vi "GPIOs.vi"(8 "error in (no error)":errorcluster, 11 "I2C in":refnum<class "I2C.lvclass">) -> (0 "error out":errorcluster, 1 "SDA GPIO":T1, 2 "SCL GPIO":T1, 3 "I2C out":refnum<class "I2C.lvclass">)   [LabVIEW 2020, in "CTI.lvlib" / "I2C.lvclass"]
uses:
  I2C.lvclass
  GPIO Number.ctl
  I2C.lvclass/I2C.ctl
  GPIO/GPIO.lvclass/GPIO.ctl
  GPIO/GPIO.lvclass
  CTI.lvlib
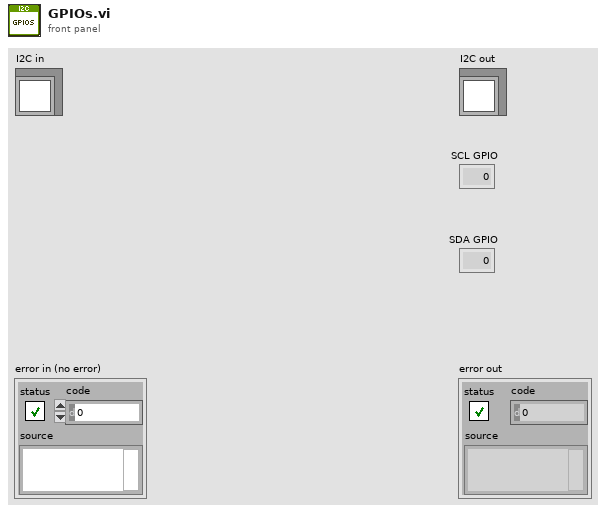
[diagram p1: front panel]
types:
  T1 = typedef "CTI.lvlib/GPIO Number.ctl" = i8
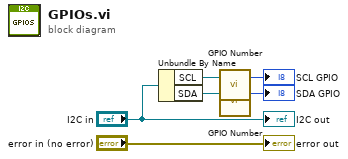
[diagram p0: block diagram]
diagram:
  n1 = Unbundle By Name("I2C in") -> ("SCL"=w4:refnum<class "GPIO.lvclass">, "SDA"=w3:refnum<class "GPIO.lvclass">)
  n2 = call "GPIO Number.vi"("GPIO in"=w4) -> ("GPIO #"=→"SCL GPIO":T1)  [unwired: 6 in]
  n3 = call "GPIO Number.vi"("GPIO in"=w3) -> ("GPIO #"=→"SDA GPIO":T1)  [unwired: 6 in]
  "error out" <- "error in (no error)"
  "I2C out" <- "I2C in"
